vi "Analysis.Calculate Yields.vi"(6 "LP Pass Cnt":i32, 7 "All Cnt":i32, 8 "FP Pass Cnt":i32, 9 "All Pass Cnt":i32, 10 "LP Cnt":i32, 11 "FP Cnt":i32) -> (3 "Yields":T1)   [LabVIEW 2024]
uses:
  Analysis.Yield Info.ctl
  Analysis.Yield Info, Item.ctl
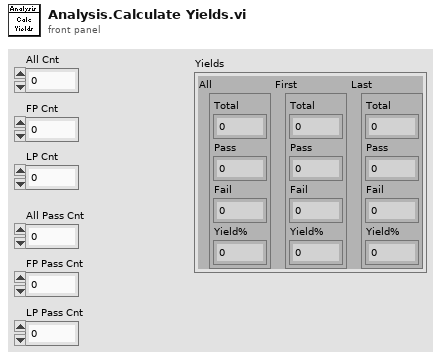
[diagram p1: front panel]
types:
  T1 = typedef "Analysis.Yield Info.ctl" = cluster{"All":T2, "First":T2, "Last":T2}
  T2 = typedef "Analysis.Yield Info, Item.ctl" = cluster{"Total":i32, "Pass":i32, "Fail":i32, "Yield%":dbl}
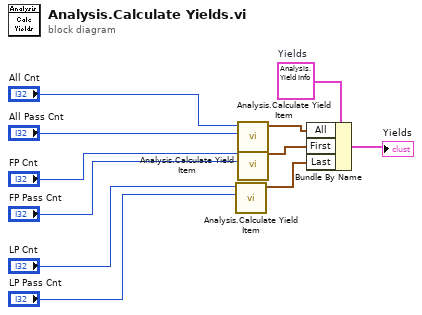
[diagram p0: block diagram]
diagram:
  w11 = T1 {"All"={"Total"=0, "Pass"=0, "Fail"=0, "Yield%"=0.0}, "First"={"Total"=0, "Pass"=0, "Fail"=0, "Yield%"=0.0}, "Last"={"Total"=0, "Pass"=0, "Fail"=0, "Yield%"=0.0}}  # Yields
  n1 = call "Analysis.Calculate Yield Item.vi"("Pass Cnt"="LP Pass Cnt", "Total Cnt"="LP Cnt") -> ("Yield"=w5:T2)  [unwired: 9 in]
  n2 = call "Analysis.Calculate Yield Item.vi"("Pass Cnt"="All Pass Cnt", "Total Cnt"="All Cnt") -> ("Yield"=w7:T2)  [unwired: 9 in]
  n3 = call "Analysis.Calculate Yield Item.vi"("Pass Cnt"="FP Pass Cnt", "Total Cnt"="FP Cnt") -> ("Yield"=w6:T2)  [unwired: 9 in]
  n4 = Bundle By Name(cluster=w11, "All"=w7, "First"=w6, "Last"=w5) -> (→"Yields":T1)
